vi "Rx Clear.vi"(8 "error in (no error)":errorcluster, 11 "Rx Session In":T1) -> (0 "error out":errorcluster)   [LabVIEW 2020, in "985x Support Addon Engine.lvlib"]
uses:
  985x Support Addon Engine.lvlib
  Types/Rx Session.ctl
  Types/FPGA Refnum.ctl
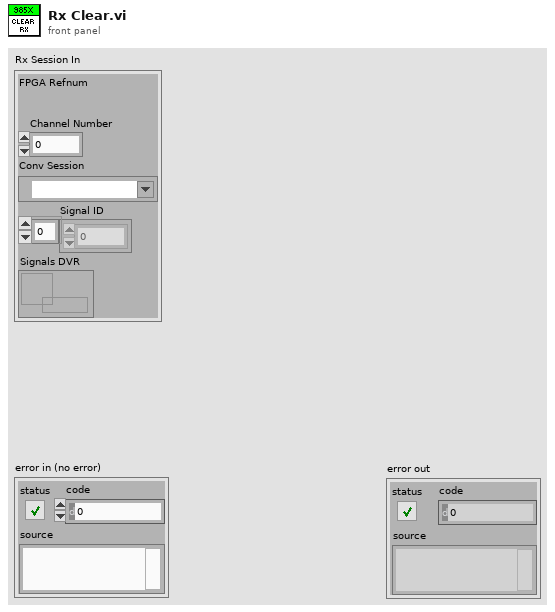
[diagram p1: front panel]
types:
  T1 = typedef "985x Support Addon Engine.lvlib/Rx Session.ctl" = cluster{"FPGA Refnum":T2, "Channel Number":u32, "Conv Session":refnum<k21>, "Signal ID":u32[], "Signals DVR":refnum<data-value>}
  T2 = typedef "985x Support Addon Engine.lvlib/FPGA Refnum.ctl" = refnum<k20>
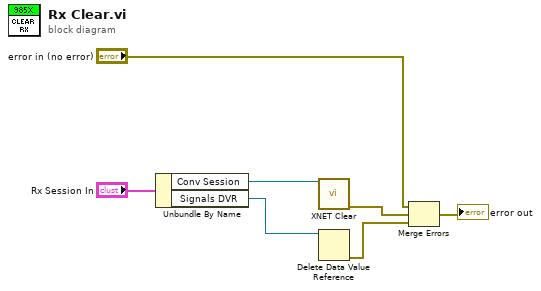
[diagram p0: block diagram]
diagram:
  n1 = Unbundle By Name("Rx Session In") -> ("Conv Session"=w6:refnum<k21>, "Signals DVR"=w3:refnum<data-value>)
  n2 = call <vilib>:"XNET Clear.vi"("session in"=w6) -> ("error out"=w5:errorcluster)  [unwired: 14 in]
  n3 = Delete Data Value Reference(data value reference=w3) -> (error out=w2:errorcluster)  [unwired: 1 in, 1 out]
  n4 = Merge Errors("error in (no error)", w5, w2) -> (→"error out":errorcluster)
